vi "TRITON_GET_VALUE.vi"(3 "error in (no error)":errorcluster, 5 "Response String":string) -> (0 "error out":errorcluster, 1 "Unit":string, 2 "Value":dbl)   [LabVIEW 2019]
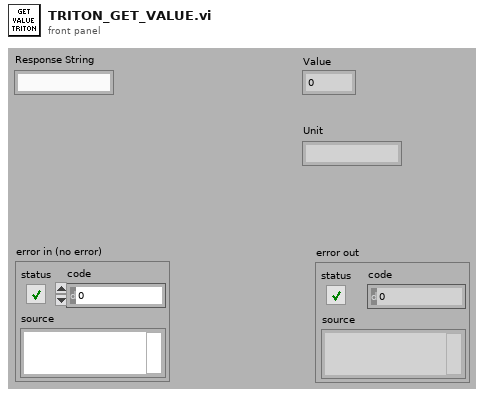
[diagram p1: front panel]
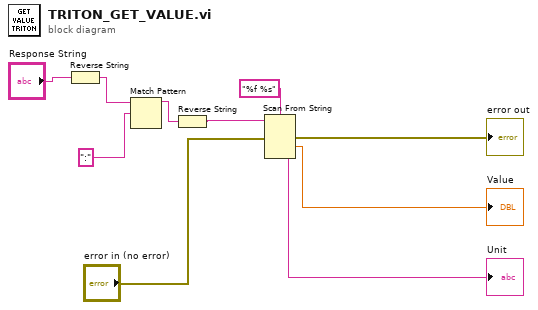
[diagram p0: block diagram]
diagram:
  n1 = Reverse String(1:"Response String") -> (0:w7:string)
  n2 = Match Pattern(string=w7, regular expression=":") -> (before substring=w5:string)  [unwired: 1 in, 3 out]
  n3 = Reverse String(1:w5) -> (0:w1:string)
  n4 = Scan From String(format string="%f %s", input string=w1, error in="error in (no error)") -> (error out=→"error out":errorcluster, output 1=→"Value":dbl, output 2=→"Unit":string)  [unwired: 3 in, 2 out]
